vi "Open Log.vi"(8 "error in (no error)":errorcluster, 11 "AMS Gas in":refnum<class "AMS Gas.lvclass">) -> (0 "error out":errorcluster, 3 "AMS Gas out":refnum<class "AMS Gas.lvclass">)   [LabVIEW 2015, in "AMS UI.lvlib" / "AMS Gas.lvclass"]
uses:
  AMS Gas.lvclass
  AMS Gas.lvclass/AMS Gas.ctl
  <vilib>/ActorFramework/Message Enqueuer/Message Enqueuer.lvclass/Message Enqueuer.ctl
  <vilib>/ActorFramework/Message Enqueuer/Enqueue.vi
  <vilib>/ActorFramework/Message Priority Queue/Priority Enqueue.vi
  eActor Messages/Open Core FP Msg/Open Core FP Msg.lvclass
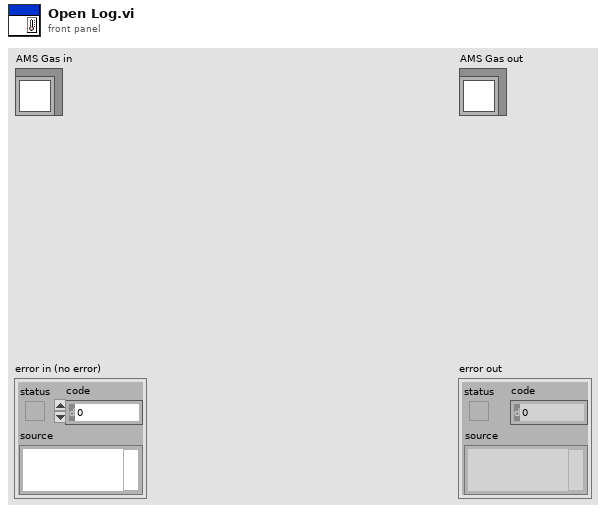
[diagram p1: front panel]
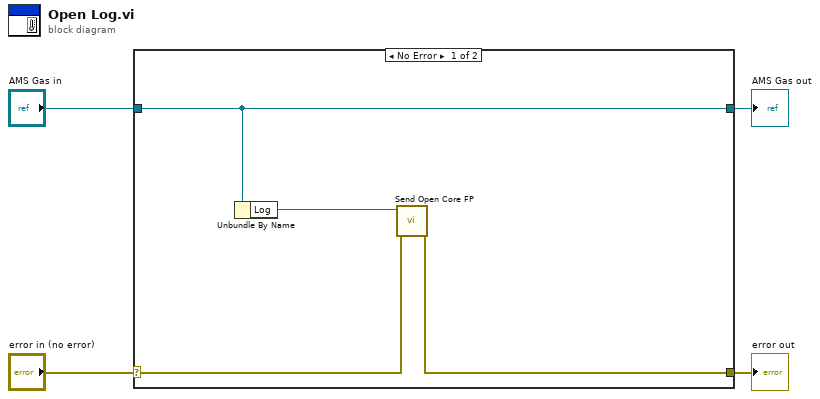
[diagram p0: block diagram]
diagram:
  n1 = case shown="No Error" "error in (no error)" {
    selector: "error in (no error)" -> [w6 w10]
    tunnel: [w5 w10] -> w3
    tunnel: [w8 w9] -> w1
    tunnel: "AMS Gas in" -> [w8 w9]
    frame No Error {
      n2 = Unbundle By Name(w8) -> ("Log"=w7:refnum<class "Message Enqueuer.lvclass">)
      n3 = call "Send Open Core FP.vi"("error in (no error)"=w6, "Message Enqueuer"=w7) -> ("error out"=w5:errorcluster)  [unwired: 8 in, 1 out]
    }
    frame Error {
    }
  }
  "error out" <- w3
  "AMS Gas out" <- w1
